vi "stage_rotary_setup.vi"(6 "serial-numbers":string[](array[string]), 8 "error_in":errorcluster, 9 "stage-select":T1(ring), 10 "ch2_ref_in":refnum<k24>, 11 "ch1_ref_in":refnum<k24>) -> (0 "ch2_error":errorcluster, 1 "ch1_error":errorcluster, 2 "ch2_ref":refnum<k24>, 3 "ch1_ref":refnum<k24>, 4 "ch2_device":refnum<k24>, 5 "ch1_device":refnum<k24>)   [LabVIEW 2024]
uses:
  O:/DSG/Tyler/EIC/DIRC/daq/automated/Thorlabs.MotionControl.Controls.dll
  Thorlabs.MotionControl.Controls.dll
  O:/DSG/Tyler/EIC/DIRC/daq/automated/Thorlabs.MotionControl.Benchtop.StepperMotorCLI.dll
  Thorlabs.MotionControl.Benchtop.StepperMotorCLI.dll
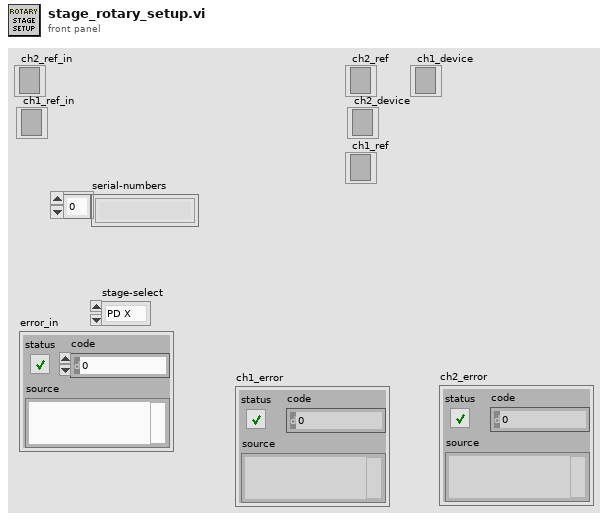
[diagram p1: front panel]
types:
  T1 = enum16{"PD X", "PD Y", "Bar X", "Bar Y", "Rotary"}
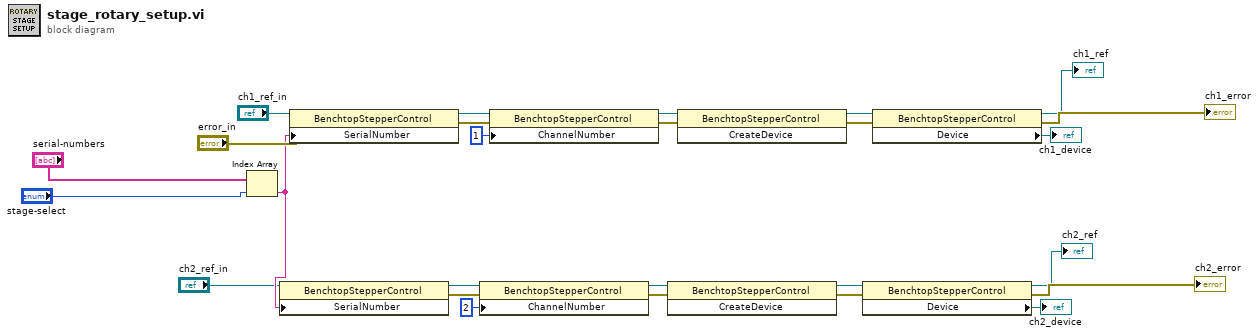
[diagram p0: block diagram]
diagram:
  n1 = Index Array(array="serial-numbers", index="stage-select") -> (element=w11:string)
  n2 = property class="BenchtopStepperControl"(reference="ch2_ref_in", "SerialNumber"=w11) -> (reference out=w15:refnum<k24>, error out=w8:errorcluster)  [unwired: 1 in]
  n3 = property class="BenchtopStepperControl"(reference="ch1_ref_in", error in="error_in", "SerialNumber"=w11) -> (reference out=w23:refnum<k24>, error out=w10:errorcluster)
  n4 = property class="BenchtopStepperControl"(reference=w15, error in=w8, "ChannelNumber"=2) -> (reference out=w16:refnum<k24>, error out=w7:errorcluster)
  n5 = property class="BenchtopStepperControl"(reference=w23, error in=w10, "ChannelNumber"=1) -> (reference out=w19:refnum<k24>, error out=w9:errorcluster)
  n6 = invoke class="BenchtopStepperControl" method="CreateDevice"(reference=w16, error in=w7) -> (reference out=w14:refnum<k24>, error out=w13:errorcluster)  [unwired: 1 in, 1 out]
  n7 = invoke class="BenchtopStepperControl" method="CreateDevice"(reference=w19, error in=w9) -> (reference out=w24:refnum<k24>, error out=w25:errorcluster)  [unwired: 1 in, 1 out]
  n8 = property class="BenchtopStepperControl"(reference=w14, error in=w13) -> (reference out=→"ch2_ref":refnum<k24>, error out=→"ch2_error":errorcluster, "Device"=→"ch2_device":refnum<k24>)
  n9 = property class="BenchtopStepperControl"(reference=w24, error in=w25) -> (reference out=→"ch1_ref":refnum<k24>, error out=→"ch1_error":errorcluster, "Device"=→"ch1_device":refnum<k24>)
